vi "process_watchdog.vi"() -> ()   [LabVIEW 2011, in "Fiberscope_library.lvlib"]
uses:
  Fiberscope_library.lvlib
  typedefs/element_images_cluster.ctl
  typedefs/element_streams_cluster.ctl
  typedefs/feedback_to_watchdog.ctl
  typedefs/feedback_from_process_enum.ctl
  globals/global_exit.vi
panel:
  out "Flush":bool
  out "Command/feedback history":i32(listbox)
  out "error out":errorcluster
  out "Averager -> Storage":bool
  out "#":i32
  out "Averager->Display":bool
  out "Pixelmapper->Averager":bool
  out "DAQ->Pixelmapper":bool
  out "#":i32
  out "#":i32
  out "#":i32
  in  "error in":errorcluster
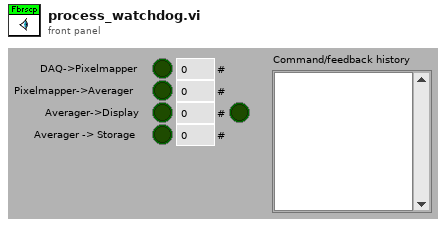
[diagram p1: front panel]
types:
  T1 = typedef "Fiberscope_library.lvlib/feedback_to_watchdog.ctl" = cluster{"Feedback_from_process_enum":T2, "Process_name":string}
  T2 = typedef "Fiberscope_library.lvlib/feedback_from_process_enum.ctl" = enum16{"Has_initialised", "Changed_parameters", "Has_started", "Has_stopped", "Has_quitted", "Is_running", "Has_finished", "Custom"}
  T3 = typedef "Fiberscope_library.lvlib/element_streams_cluster.ctl" = cluster{"Streams_array":dbl[][], "#channels":i32, "Last element?":bool, "Forth (1) or back (0)?":bool}
  T4 = typedef "Fiberscope_library.lvlib/element_images_cluster.ctl" = cluster{"Images_array":dbl[][][], "#channels":i32, "Last element?":bool}
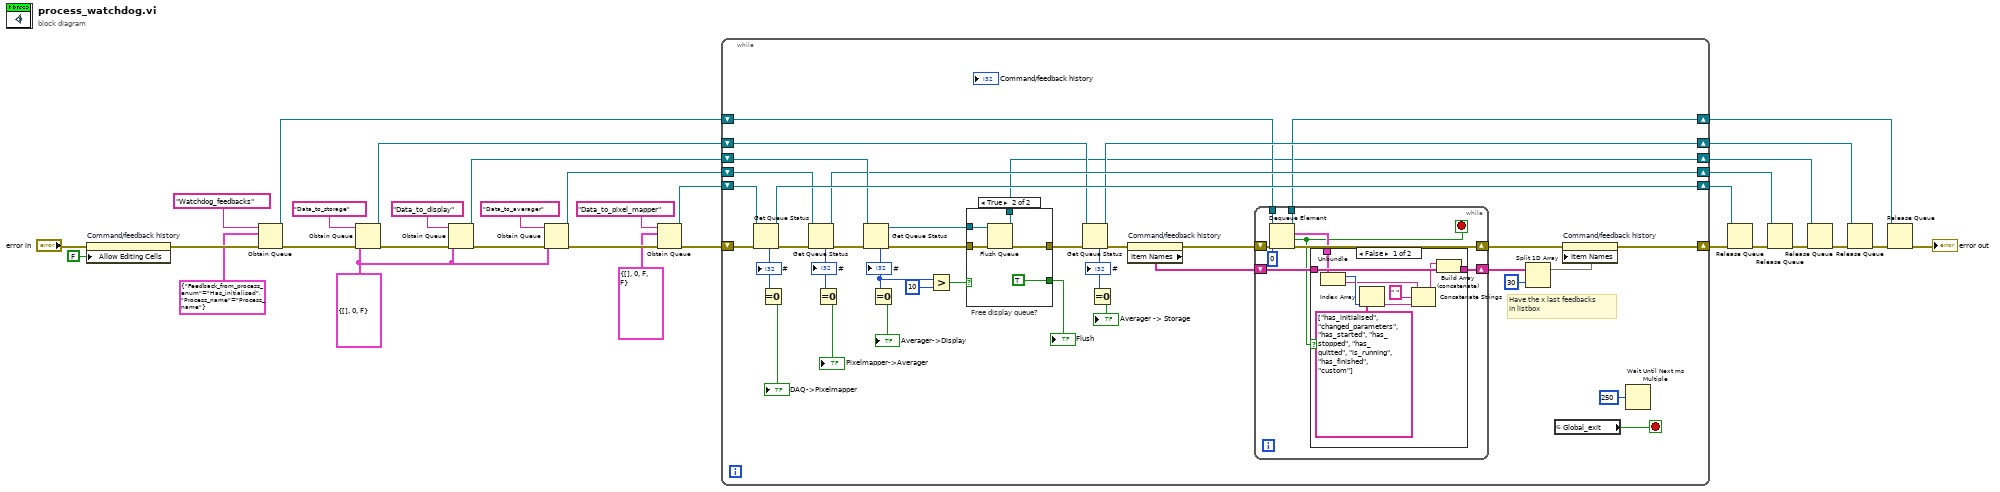
[diagram p0: block diagram]
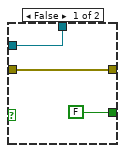
[diagram p2: hidden frame]
diagram:
  w18 = T4 {"Images_array"=[], "#channels"=0, "Last element?"=FALSE} ("Element_images_cluster")
  n1 = property on="Command/feedback history" class="LstBox (strict)"(error in="error in", "Allow Editing Cells"=FALSE) -> (error out=w10:errorcluster)  [unwired: 1 in, 1 out]
  n2 = Obtain Queue(name (unnamed)="Watchdog_feedbacks", element data type=T1 {"Feedback_from_process_enum"=enum."Has_initialised", "Process_name"="Process_name"}, error in (no error)=w10) -> (queue out=w14:refnum<queue>, error out=w16:errorcluster)  [unwired: 2 in, 1 out]
  n3 = Obtain Queue(name (unnamed)="Data_to_storage", element data type=w18, error in (no error)=w16) -> (queue out=w20:refnum<queue>, error out=w22:errorcluster)  [unwired: 2 in, 1 out]
  n4 = Obtain Queue(name (unnamed)="Data_to_display", element data type=w18, error in (no error)=w22) -> (queue out=w31:refnum<queue>, error out=w29:errorcluster)  [unwired: 2 in, 1 out]
  n5 = Obtain Queue(name (unnamed)="Data_to_averager", element data type=w18, error in (no error)=w29) -> (queue out=w28:refnum<queue>, error out=w26:errorcluster)  [unwired: 2 in, 1 out]
  n6 = Obtain Queue(name (unnamed)="Data_to_pixel_mapper", element data type=T3 {"Streams_array"=[], "#channels"=0, "Last element?"=FALSE, "Forth (1) or back (0)?"=FALSE} ("Element_streams_cluster"), error in (no error)=w26) -> (queue out=w24:refnum<queue>, error out=w25:errorcluster)  [unwired: 2 in, 1 out]
  n7 = while {
    shift-right: [w48] -> w23
    shift-left: w25 -> [w67]
    shift-right: [w35] -> w2
    shift-left: w31 -> [w61]
    shift-right: [w60] -> w3
    shift-left: w28 -> [w62]
    shift-right: [w65] -> w17
    shift-left: w24 -> [w66]
    shift-right: [w53] -> w1
    shift-left: w20 -> [w54]
    shift-right: [w49] -> w13
    shift-left: w14 -> [w50]
    stop <- w68 stop-if-true
    # "Have the x last feedbacks\nin listbox"
    n8 = Get Queue Status(queue=w66, error in (no error)=w67) -> (queue out=w65:refnum<queue>, error out=w64:errorcluster, # elements in queue=w59:i32)  [unwired: 1 in, 5 out]
    "#" <- w59
    n9 = Equal To 0?(x=w59) -> (x = 0?=→"DAQ->Pixelmapper":bool)
    n10 = Get Queue Status(queue=w62, error in (no error)=w64) -> (queue out=w60:refnum<queue>, error out=w63:errorcluster, # elements in queue=w58:i32)  [unwired: 1 in, 5 out]
    "#" <- w58
    n11 = Equal To 0?(x=w58) -> (x = 0?=→"Pixelmapper->Averager":bool)
    n12 = Get Queue Status(queue=w61, error in (no error)=w63) -> (queue out=w36:refnum<queue>, error out=w38:errorcluster, # elements in queue=w40:i32)  [unwired: 1 in, 5 out]
    "#" <- w40
    n13 = Equal To 0?(x=w40) -> (x = 0?=→"Averager->Display":bool)
    n14 = Greater?(x=w40, y=10) -> (0:w34:bool)
    n15 = case "Free display queue?" shown="True" w34 {
      tunnel: w38 -> [w72 w77]
      tunnel: [w72 w76] -> w37
      tunnel: w36 -> [w71 w75]
      tunnel: [w71 w74] -> w35
      tunnel: [FALSE ("Flush") TRUE ("Flush")] -> w33
      frame False {
      }
      frame True {
        n16 = Flush Queue(queue=w75, error in (no error)=w77) -> (queue out=w74:refnum<queue>, error out=w76:errorcluster)  [unwired: 1 out]
      }
    }
    "Flush" <- w33
    n17 = Get Queue Status(queue=w54, error in (no error)=w37) -> (queue out=w53:refnum<queue>, error out=w47:errorcluster, # elements in queue=w52:i32)  [unwired: 1 in, 5 out]
    "#" <- w52
    n18 = Equal To 0?(x=w52) -> (x = 0?=→"Averager -> Storage":bool)
    n19 = property on="Command/feedback history" class="LstBox (strict)"(error in=w47) -> (error out=w46:errorcluster, "Item Names"=w44:string[])  [unwired: 1 in, 1 out]
    n20 = while {
      tunnel: w50 -> [w86]
      tunnel: [w85] -> w49
      shift-right: [w81] -> w43
      shift-left: w44 -> [w82]
      shift-right: [w83] -> w45
      shift-left: w46 -> [w84]
      stop <- w78 stop-if-true
      n21 = Dequeue Element(queue=w86, timeout in ms (-1)=0, error in (no error)=w84) -> (queue out=w85:refnum<queue>, element=w80:T1, timed out?=w78:bool, error out=w83:errorcluster)
      n22 = case shown="False" w78 {
        tunnel: w82 -> [w94 w96]
        tunnel: [w93 w96] -> w81
        tunnel: w80 -> [w92 _]
        frame False {
          n23 = Unbundle(w92) -> ("Feedback_from_process_enum"=w91:T2, "Process_name"=w89:string)
          n24 = Index Array(array=string[] ["has_initialised", "changed_parameters", "has_started", "has_stopped", "has_quitted", "is_running", "has_finished", "custom"], index=w91) -> (element=w88:string)
          n25 = Concatenate Strings(w89, " " ("string"), w88) -> (w90:string)
          n26 = Build Array (concatenate)(w90, w94) -> (w93:string[])
        }
        frame True {
        }
      }
    }
    n27 = Split 1D Array(array=w43, index=30) -> (first subarray=w41:string[])  [unwired: 1 out]
    n28 = global read "global_exit.vi" "Global_exit"() -> (w68:bool)
    n29 = property on="Command/feedback history" class="LstBox (strict)"(error in=w45, "Item Names"=w41) -> (error out=w48:errorcluster)  [unwired: 1 in, 1 out]
    n30 = Wait Until Next ms Multiple(millisecond multiple=u32 250) -> ()  [unwired: 1 out]
  }
  n31 = Release Queue(queue=w17, error in (no error)=w23) -> (error out=w7:errorcluster)  [unwired: 1 in, 2 out]
  n32 = Release Queue(queue=w3, error in (no error)=w7) -> (error out=w6:errorcluster)  [unwired: 1 in, 2 out]
  n33 = Release Queue(queue=w2, error in (no error)=w6) -> (error out=w5:errorcluster)  [unwired: 1 in, 2 out]
  n34 = Release Queue(queue=w1, error in (no error)=w5) -> (error out=w4:errorcluster)  [unwired: 1 in, 2 out]
  n35 = Release Queue(queue=w13, error in (no error)=w4) -> (error out=→"error out":errorcluster)  [unwired: 1 in, 2 out]
